vi "hmi_browse_update_version.vi"(8 "error in (no error)":errorcluster, 11 "update_version_vi":string) -> (0 "error out":errorcluster, 3 "selected path":path)   [LabVIEW 2015, in "lv-builder-default.lvlib"]
uses:
  lv-builder-default.lvlib
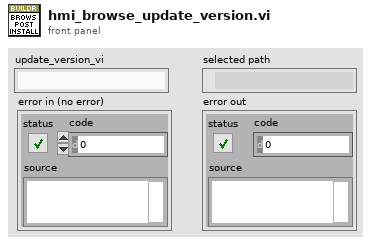
[diagram p1: front panel]
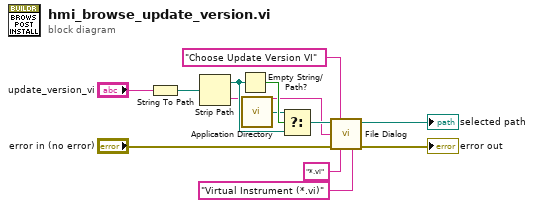
[diagram p0: block diagram]
diagram:
  n1 = String To Path(string="update_version_vi") -> (path=w9:path)
  n2 = Strip Path(path=w9) -> (stripped path=w5:path, name=w3:string)
  n3 = Empty String/Path?(string/path=w5) -> (empty?=w10:bool)
  n4 = call <vilib>:"Application Directory.vi"() -> ("Application Directory"=w7:path)
  n5 = Select(t=w7, s=w10, f=w5) -> (s? t:f=w11:path)
  n6 = call "File Dialog"("start path"=w11, "prompt"="Choose Update Version VI" ("description"), "default name"=w3, "error in"="error in (no error)", "pattern (all files)"="*.vi" ("filter"), "pattern label"="Virtual Instrument (*.vi)" ("filter")) -> ("selected path"=→"selected path":path, "error out"=→"error out":errorcluster)  [unwired: 6 in, 2 out]
